vi "DriveTuningGlobals.vi"() -> ()   [LabVIEW 2023]
panel:
  out "DriveKsKvMotorDmd":dbl
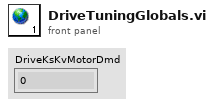
[diagram p1: front panel]
diagram:
